vi "Convert Array to String.vi"(0 "StringArrayIn":string[](array[string])=["", "", "", "", "", ""], 1 "Type":T1(ring), 2 "Delimiter(comma)":string=",", 5 "I32ArrayIn":i32[](array[numeric])=[101, 102, 103, 104, 105, 106], 7 "SglArrayIn":sgl[](array[numeric])=[101.0, 102.0, 103.0, 104.0, 105.0, 106.0] format="%.2f", 9 "DblArrayIn":dbl[](array[numeric])=[101.0, 102.0, 103.0, 104.0, 105.0, 106.0] format="%.2f", 11 "BooleanArrayIn":bool[](array[boolean])=[FALSE, FALSE, FALSE, FALSE, FALSE, FALSE], 12 "U32ArrayIn":u32[](array[numeric])=[101, 102, 103, 104, 105, 106], 13 "PathArrayIn":path[](array[path])) -> (8 "StringOut":string="101,102,103,104,105,106")   [LabVIEW 2013]
doc: "Converts an input array selected by 'Type' to a string separated by the 'Delimiter' (def = comma). Typically used with file output to store values on a single ASCII line. The input array may be of any size; the output string reflects the array size. AutoCon, 11/98"
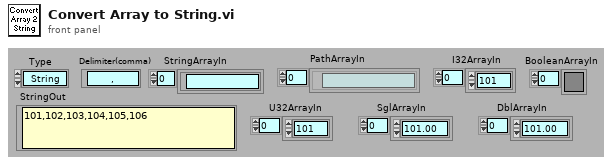
[diagram p1: front panel]
types:
  T1 = enum16{"String", "I32", "Sgl", "Dbl", "Boolean", "U32", "Path"}
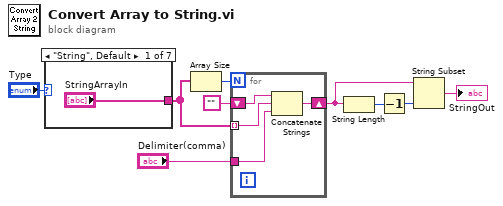
[diagram p0: block diagram]
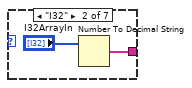
[diagram p2: hidden frame]
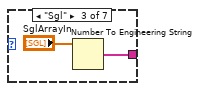
[diagram p3: hidden frame]
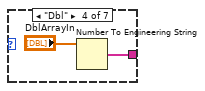
[diagram p4: hidden frame]
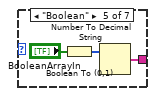
[diagram p5: hidden frame]
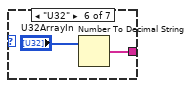
[diagram p6: hidden frame]
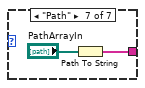
[diagram p7: hidden frame]
diagram:
  n1 = case shown="\"String\", Default" "Type" {
    tunnel: ["StringArrayIn" w12 w14 w16 w19 w21 w22] -> w3
    frame "String", Default {
    }
    frame "I32" {
      n2 = Number To Decimal String(number="I32ArrayIn") -> (decimal integer string=w12:string[])  [unwired: 1 in]
    }
    frame "Sgl" {
      n3 = Number To Engineering String(4:"SglArrayIn") -> (0:w14:string[])  [unwired: 3 in]
    }
    frame "Dbl" {
      n4 = Number To Engineering String(4:"DblArrayIn") -> (0:w16:string[])  [unwired: 3 in]
    }
    frame "Boolean" {
      n5 = Boolean To (0,1)(Boolean="BooleanArrayIn") -> (0, 1=w18:i16[])
      n6 = Number To Decimal String(number=w18) -> (decimal integer string=w19:string[])  [unwired: 1 in]
    }
    frame "U32" {
      n7 = Number To Decimal String(number="U32ArrayIn") -> (decimal integer string=w21:string[])  [unwired: 1 in]
    }
    frame "Path" {
      n8 = Path To String(path="PathArrayIn") -> (string=w22:string[])
    }
  }
  n9 = Array Size(array=w3) -> (size(s)=w9:i32)
  n10 = for {
    N: w9 -> [_]
    tunnel: w3 -> [w24] mode=indexing
    shift-right: [w26] -> w7
    shift-left: "" -> [w27]
    tunnel: "Delimiter(comma)" -> [w25]
    n11 = Concatenate Strings(w27, w24, w25) -> (w26:string)
  }
  n12 = String Length(string=w7) -> (length=w6:i32)
  n13 = Decrement(x=w6) -> (x-1=w5:i32)
  n14 = String Subset(string=w7, length (rest)=w5) -> (substring=→"StringOut":string)  [unwired: 1 in]
